vi "HelloWorld.vi"() -> ()   [LabVIEW 2022 SP3]
uses:
  <vilib>/express/express analysis/Spectral/Block/exnSpectralBlock spectral measurements power poly.vi
  <vilib>/express/express analysis/Spectral/Block/exnSpectralBlock spectral measurements power DDT.vi
  <vilib>/express/express analysis/Spectral/XNode/ExpressSpectralMeasurementsBlockNode.xnode
panel:
  in  "Save Button":bool
  in  "Tab Control":enum32{"temperature", "sound", "Spectrum"}(tab)
  out "Temperature Waveform Chart":dbl(graph)
  out "Sound Graph":dynamicdata(graph)
  out "Spectrum":dynamicdata(graph)
  out "Thermometer":dbl(slide) scale=10.0..100.0
  in  "Temperature\nmaximum":dbl
  in  "stop":bool
  out "Boolean":bool
  out "Temperature":dbl
  in  "Temperature\nAdjuster":dbl(knob) scale=0.0..10.0
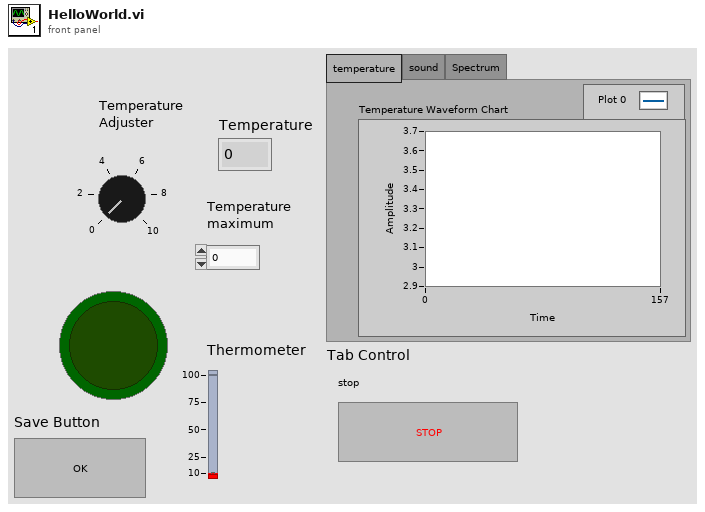
[diagram p1: front panel]
types:
  T1 = cluster{"averaging mode":u16, "weighting mode":u16, "number of averages":u32}
  T2 = cluster{"dB On (F)":bool, "unwrap phase (F)":bool, "convert to degree (F)":bool}
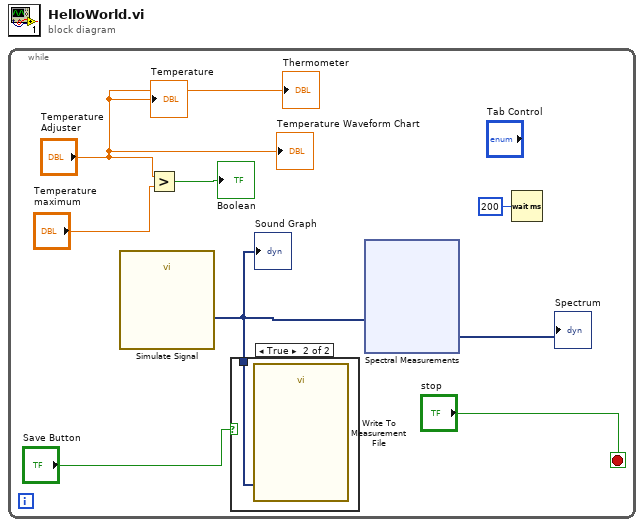
[diagram p0: block diagram]
diagram:
  n1 = while {
    stop <- "stop" stop-if-true
    n2 = call "Simulate Signal"() -> ("Sine"=w3:dynamicdata)  [unwired: 14 in, 1 out]
    "Sound Graph" <- w3
    n3 = Greater?(x="Temperature\nAdjuster", y="Temperature\nmaximum") -> (0:→"Boolean":bool)
    n4 = case shown="True" "Save Button" {
      tunnel: w3 -> [_ w9]
      frame False {
      }
      frame True {
        n5 = call "Write To Measurement File"("Signals"=w9) -> ()  [unwired: 16 in, 3 out]
      }
    }
    n6 = xnode "Spectral Measurements"("Signals"=w3) -> ("Power Spectrum"=→"Spectrum":dynamicdata)  [unwired: 1 in, 1 out]
    n7 = Wait (ms)(milliseconds to wait=u32 200) -> ()  [unwired: 1 out]
    "Temperature" <- "Temperature\nAdjuster"
    "Temperature Waveform Chart" <- "Temperature\nAdjuster"
    "Thermometer" <- "Temperature\nAdjuster"
  }
